vi "clock_gettime.vi"(8 "error in (no error)":errorcluster, 11 "clock id (monotonic)":T2=enum."Monotonic") -> (0 "error out":errorcluster, 3 "timespec":T1)   [LabVIEW 2013, in "Linux RT Utilities.lvlib"]
uses:
  Linux RT Utilities.lvlib
  Controls/Public/C Enums/clockid_t.ctl
  Controls/Public/C Structs/timespec_64.ctl
  Controls/Public/C Structs/timespec_32.ctl
  <vilib>/Utility/error.llb/Error Cluster From Error Code.vi
  <vilib>/NI/NI Linux RT Errno/Public/VIs/Get LV Error Info from Errno.vi
  <vilib>/NI/NI Linux RT Errno/Linux Errno.lvlib
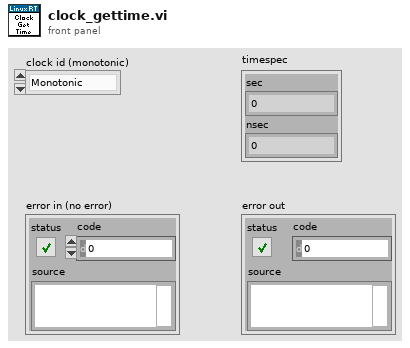
[diagram p1: front panel]
types:
  T1 = typedef "Linux RT Utilities.lvlib/timespec_64.ctl" = cluster{"sec":u64, "nsec":u64}
  T2 = typedef "Linux RT Utilities.lvlib/clockid_t.ctl" = enum16{"Realtime", "Monotonic"}
  T3 = typedef "Linux RT Utilities.lvlib/timespec_32.ctl" = cluster{"sec":u32, "nsec":u32}
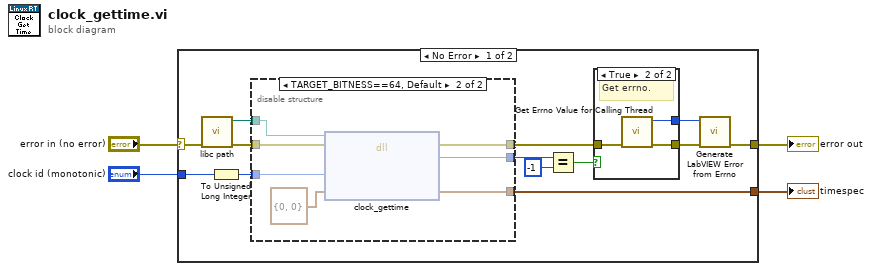
[diagram p0: block diagram]
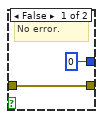
[diagram p2: hidden frame]
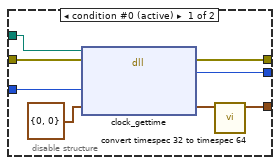
[diagram p3: hidden frame]
diagram:
  n1 = case shown="No Error" "error in (no error)" {
    selector: "error in (no error)" -> [w7 w38]
    tunnel: [w15 w38] -> w4
    tunnel: [w17 _] -> w1
    tunnel: "clock id (monotonic)" -> [w16 _]
    frame No Error {
      n2 = call "libc path.vi"("error in (no error)"=w7) -> ("error out"=w6:errorcluster, "Path"=w5:path)  [unwired: 9 in]
      n3 = To Unsigned Long Integer(number=w16) -> (unsigned 32bit integer=w14:u32)
      n4 = disable-structure shown="TARGET_BITNESS==64, Default" {
        disable-tunnel: w6 -> [w24 w37]
        disable-tunnel: w14 -> [w30 w36]
        disable-tunnel: [w27 w33] -> w17
        disable-tunnel: [w26 w35] -> w11
        disable-tunnel: [w25 w34] -> w13
        disable-tunnel: w5 -> [w23 w31]
        frame condition #0 (active) {
          n5 = dll-call lib="lib/libc.so.6" fn="clock_gettime"(path in=w23, error in=w24, "clock_id"=w30, "timespec"=T3 {"sec"=0, "nsec"=0}) -> (error out=w26:errorcluster, "status"=w25:i32, "timespec"=w28:T3)  [unwired: 2 in, 1 out]
          n6 = call "convert timespec 32 to timespec 64.vi"("timespec 32"=w28) -> ("timespec 64"=w27:T1)  [unwired: 10 in]
        }
        frame condition #1 {
          n7 = dll-call lib="lib/libc.so.6" fn="clock_gettime"(path in=w31, error in=w37, "clock_id"=w36, "timespec"=T1 {"sec"=0, "nsec"=0}) -> (error out=w35:errorcluster, "status"=w34:i32, "timespec"=w33:T1)  [unwired: 2 in, 1 out]
        }
      }
      n8 = Equal?(x=w13, y=-1) -> (x = y?=w10:bool)
      n9 = case shown="True" w10 {
        tunnel: w11 -> [w19 w22]
        tunnel: [w19 w21] -> w9
        tunnel: [0 ("errno") w20] -> w8
        frame False {
          # "No error."
        }
        frame True {
          # "Get errno."
          n10 = call <vilib>:"Get Errno Value for Calling Thread.vi"("error in (no error)"=w22) -> ("error out"=w21:errorcluster, "errno"=w20:i32)  [unwired: 9 in]
        }
      }
      n11 = call <vilib>:"Generate LabVIEW Error from Errno.vi"("error in (no error)"=w9, "errno"=w8) -> ("error out"=w15:errorcluster)  [unwired: 9 in]
    }
    frame Error {
    }
  }
  "error out" <- w4
  "timespec" <- w1
